vi "Get SGL.vi"(8 "error in (no error)":errorcluster, 9 "Data Type (default value)":sgl, 10 "Offset":i32, 11 "JSON":string) -> (0 "error out":errorcluster, 1 "Number":sgl format="%.2f", 2 "Offset past match":i32)   [LabVIEW 2017, in "JSONtext.lvlib"]
uses:
  JSONtext.lvlib
  String Subset.vi
  Parsing/Advance past Number.vi
  Parsing/Parsing Error.vi
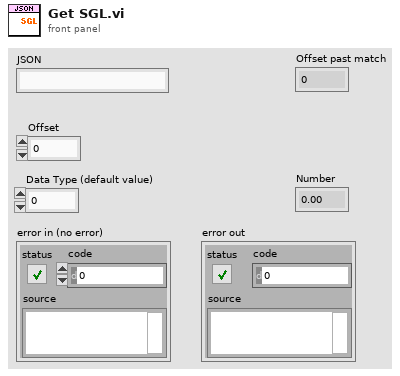
[diagram p1: front panel]
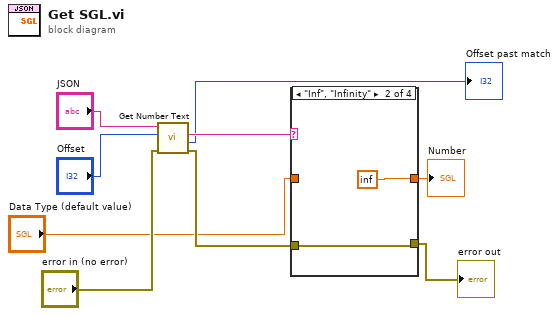
[diagram p0: block diagram]
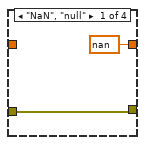
[diagram p2: hidden frame]
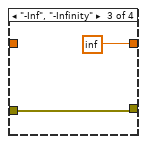
[diagram p3: hidden frame]
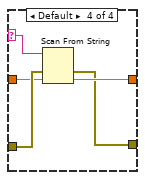
[diagram p4: hidden frame]
diagram:
  n1 = call "Get Number Text.vi"("error in (no error)"="error in (no error)", "Offset"="Offset", "JSON"="JSON") -> ("error out"=w6:errorcluster, "Offset past match"=→"Offset past match":i32, "Number Text"=w4:string)  [unwired: 5 in, 1 out]
  n2 = case shown="\"Inf\", \"Infinity\"" w4 {
    selector: w4 -> [_ _ _ w16]
    tunnel: [sgl nan ("default value 1") sgl inf ("default value 1") sgl inf ("default value 1") w20] -> w3
    tunnel: w6 -> [w11 w12 w14 w19]
    tunnel: [w11 w12 w14 w18] -> w5
    tunnel: "Data Type (default value)" -> [_ _ _ w17]
    frame "NaN", "null" {
    }
    frame "Inf", "Infinity" {
    }
    frame "-Inf", "-Infinity" {
    }
    frame Default {
      n3 = Scan From String(input string=w16, error in=w19, default 1=w17) -> (error out=w18:errorcluster, output 1=w20:sgl)  [unwired: 2 in, 2 out]
    }
  }
  "error out" <- w5
  "Number" <- w3
